vi "Wait_No_cDAQ.vi"(9 "PS VISA in":refnum<visa-resource-name>, 11 "PS error in":errorcluster caption="PS error in (no error)", 12 "Wait Filepath":path=path "C:/Users/ga11/Desktop/VI/results/3PtestChrgRest.lvm" caption="Filename", 13 "Wait time":dbl) -> (10 "PS Visa Out":refnum<visa-resource-name>, 15 "PS error out":errorcluster)   [LabVIEW 2020]
uses:
  Drivers-NHR-9200/NHR/Public/Data/Low Level/Fetch (Ave Voltage).vi
  Drivers-NHR-9200/NHR/NH Research Regenerative Test Series.lvlib
panel:
  out "Ave Current (A)":dbl
  out "Ave Voltage (V)":dbl
  out "WaitElapsed Time (s)":i32 caption="Elapsed Time (s)"
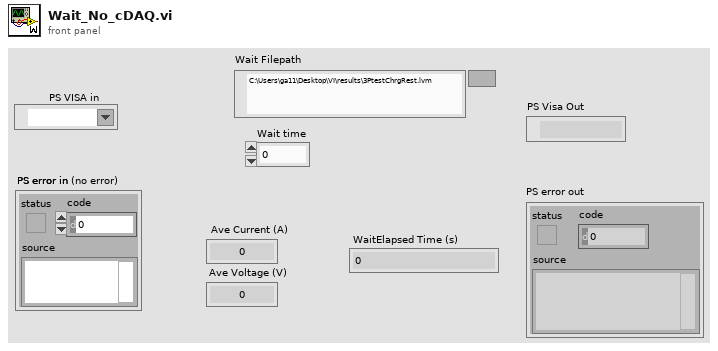
[diagram p1: front panel]
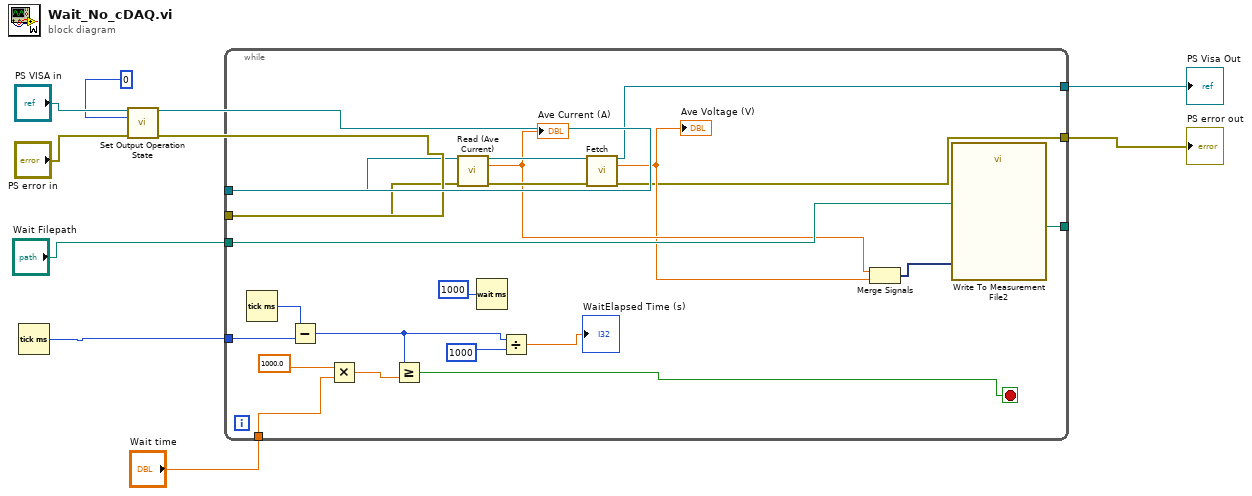
[diagram p0: block diagram]
diagram:
  n1 = Tick Count (ms)() -> (millisecond timer value=w9:u32)
  n2 = call "Set Output Operation State.vi"("VISA resource name"="PS VISA in", "Mode (0: Off)"=0, "error in (no error)"="PS error in") -> ("VISA resource name out"=w2:refnum<visa-resource-name>, "error out"=w1:errorcluster)  [unwired: 11 in]
  n3 = while {
    tunnel: w2 -> [w29]
    tunnel: w1 -> [w28]
    tunnel: "Wait time" -> [w24]
    tunnel: [w21] -> _
    tunnel: w9 -> [w20]
    tunnel: "Wait Filepath" -> [w19]
    tunnel: [w12] -> w5
    tunnel: [w11] -> w4
    stop <- w25 stop-if-true
    n4 = Tick Count (ms)() -> (millisecond timer value=w26:u32)
    n5 = Subtract(x=w26, y=w20) -> (x-y=w18:u32)
    n6 = Multiply(x=1000.0, y=w24) -> (x*y=w22:dbl)
    n7 = Greater Or Equal?(x=w18, y=w22) -> (x >= y?=w25:bool)
    n8 = call "Read (Ave Current).vi"("VISA resource name"=w29, "error in (no error)"=w28) -> ("VISA resource name out"=w30:refnum<visa-resource-name>, "Ave Current (A)"=w15:dbl, "error out"=w31:errorcluster)  [unwired: 11 in]
    "Ave Current (A)" <- w15
    n9 = Wait (ms)(milliseconds to wait=1000) -> ()  [unwired: 1 out]
    n10 = Divide(x=w18, y=1000) -> (x/y=→"WaitElapsed Time (s)":dbl)
    n11 = call-poly "Fetch.vi"("VISA resource name"=w30, "error in (no error)"=w31) -> ("VISA resource name out"=w12:refnum<visa-resource-name>, "Ave Voltage (V)"=w13:dbl, "error out"=w11:errorcluster)  [unwired: 11 in]
    "Ave Voltage (V)" <- w13
    n12 = Merge Signals "Merge Signals"(w15, w13) -> (w14:dynamicdata)
    n13 = call "Write To Measurement File2"("Signals"=w14, "Filename"=w19) -> ("Filename Out"=w21:path)  [unwired: 15 in, 2 out]
  }
  "PS Visa Out" <- w5
  "PS error out" <- w4
